vi "Push Double Batch.vi"(8 "error in (no error)":errorcluster, 9 "Values":dbl[](array[numeric]), 10 "Timestamps":timestamp[](array[timestamp]) format="%<%x %.3X>T", 11 "Channel in":refnum<class "Channel.lvclass">) -> (0 "error out":errorcluster, 3 "Channel out":refnum<class "Channel.lvclass">)   [LabVIEW 2020, in "Nominal Streaming.lvlib" / "Channel.lvclass"]
doc: "Streams data to Nominal Core.\nAny `Not a Number` (NaN) values will be filtered out.\nReturns an error if there is a mismatch in input array sizes."
uses:
  Channel.lvclass
  Channel.lvclass/Channel.ctl
  Stream/Stream.lvclass
  Nominal Streaming/Nominal Streaming.lvlib
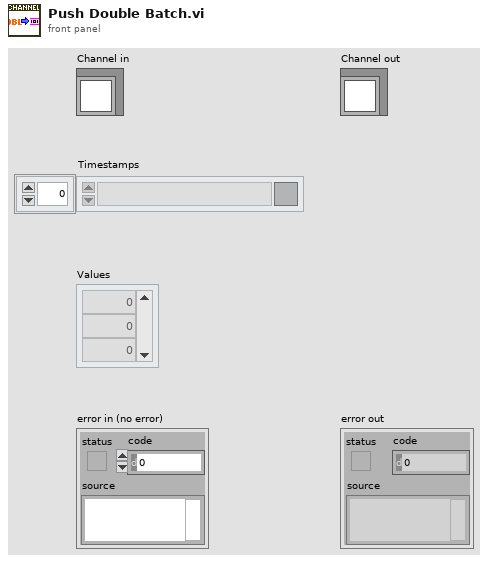
[diagram p1: front panel]
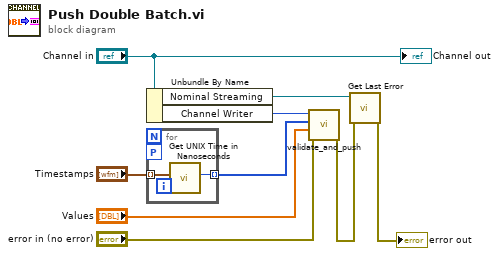
[diagram p0: block diagram]
diagram:
  n1 = Unbundle By Name("Channel in") -> ("Nominal Streaming"=w7:refnum<class "Stream.lvclass">, "Channel Writer"=w5:u64)
  n2 = for {
    tunnel: "Timestamps" -> [w11] mode=indexing
    tunnel: [w10] -> w4 mode=indexing
    workers-P: _ -> [_]
    n3 = call "Get UNIX Time in Nanoseconds.vi"("Time Stamp"=w11) -> ("UNIX Time (ns)"=w10:u64)  [unwired: 10 in]
  }
  n4 = call "validate_and_push.vi"("error in (no error)"="error in (no error)", "values"="Values", "timestamps_ns"=w4, "writer_handle"=w5) -> ("error out"=w1:errorcluster)  [unwired: 7 in]
  n5 = call "Get Last Error.vi"("error in (no error)"=w1, "Nominal Streaming in"=w7) -> ("error out"=→"error out":errorcluster)  [unwired: 8 in, 1 out]
  "Channel out" <- "Channel in"
